vi "OpenTalonDrive.vi"   [LabVIEW 2016]
uses:
  <vilib>/Rock Robotics/WPI/ThirdParty/CanMotor/TalonSRX/WPI_CANTalonSRX_APIControlMode.ctl
  <vilib>/Rock Robotics/WPI/SafetyOutput/WPI_SafetyOutputConfigMenu.ctl
  <vilib>/Rock Robotics/WPI/ThirdParty/CanMotor/TalonSRX/WPI_CANTalonSRX_APIFeedbackSelect.ctl
types:
  T1 = typedef "WPI_CANTalonSRX_APIFeedbackSelect.ctl" = enum16{"Digital Quadrature Encoder", "Analog Potentiometer", "Analog Encoder", "Count on Quad-A (Rising-Edge)", "Count on Quad-A (Falling-Edge)", "CTR Magnetic Enc (Absolute)", "CTR Magnetic Enc (Relative)", "Pulse Width"}
  T2 = typedef "WPI_SafetyOutputConfigMenu.ctl" = enum16{"Enable", "Disable"}
  T3 = typedef "WPI_CANTalonSRX_APIControlMode.ctl" = enum8{"Percent VBus", "Speed", "Position", "Slave", "Unchanged / Invalid", "Voltage Compensation", "Current", "Motion Profile", "Motion Magic"}
  T4 = typedef "WPI_MotorControlDeviceRef.ctl" = cluster{"DeviceStatus":errorcluster, "Type":T5, "PWM":cluster{"PWM Channel":T6, "DeadBand":T7}, "CAN":cluster{"Device Number":u8, "SetOutput VI Ref":variant, "GetOutput VI Ref":variant, "Enable VI Ref":variant, "Disable VI Ref":variant, "Data":variant}, "Invert":bool}
  T5 = typedef "WPI_MotorControlType.ctl" = enum16{"PWM", "CAN"}
  T6 = typedef "FPGA_DIOPWMChannel.ctl" = enum8{"PWM 0", "PWM 1", "PWM 2", "PWM 3", "PWM 4", "PWM 5", "PWM 6", "PWM 7", "PWM 8", "PWM 9", "PWM MXP 0", "PWM MXP 1", "PWM MXP 2", "PWM MXP 3", "PWM MXP 4", "PWM MXP 5", "PWM MXP 6", "PWM MXP 7", "PWM MXP 8", "PWM MXP 9", "Invalid"}
  T7 = typedef "WPI_PWMDeadband.ctl" = cluster{"Name":string, "maxPositivePwm":i32, "minPositivePwm":i32, "centerPwm":i32, "maxNegativePwm":i32, "minNegativePwm":i32, "angularRange":u16}
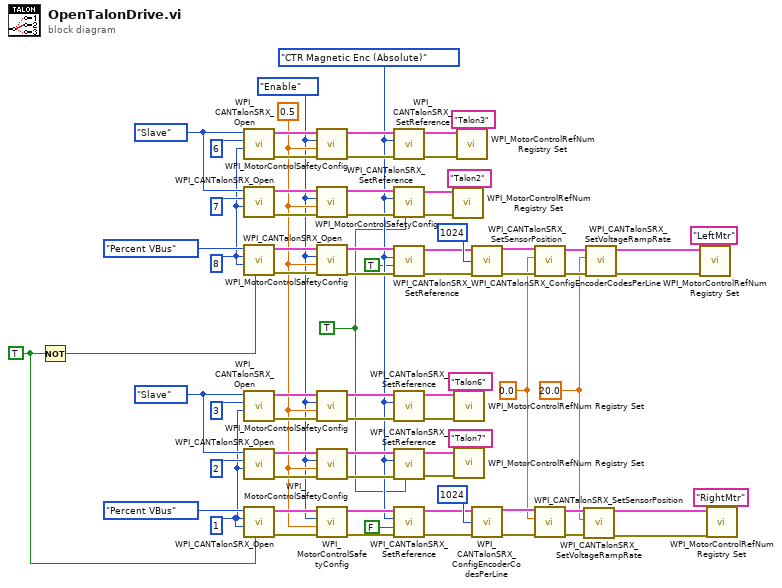
[diagram p0: block diagram]
diagram:
  w5 = 20.0 ("Throttle Ramp Rate (percent/s)")
  w14 = TRUE
  w15 = TRUE
  w30 = WPI_CANTalonSRX_APIFeedbackSelect."CTR Magnetic Enc (Absolute)" ("Feedback Reference")
  w47 = WPI_SafetyOutputConfigMenu."Enable" ("mode")
  w10 = 0.0 ("New Sensor Position")
  w17 = u8 1 ("Device Number")
  w62 = WPI_CANTalonSRX_APIControlMode."Slave" ("Control Mode")
  w48 = 0.5 ("timeout (s)")
  w16 = u8 8 ("Device Number")
  w76 = WPI_CANTalonSRX_APIControlMode."Slave" ("Control Mode")
  n1 = Not(x=w14) -> (.not. x?=w13:bool)
  n2 = call <vilib>:"WPI_CANTalonSRX_Open.vi"("Master Device Number"=w16, "Device Number"=u8 6, "Control Mode"=w76) -> ("error out"=w69:errorcluster, "CAN Talon SRX Ref"=w70:T4)  [unwired: 7 in]
  n3 = call <vilib>:"WPI_CANTalonSRX_Open.vi"("Master Device Number"=w16, "Device Number"=u8 7, "Control Mode"=w76) -> ("error out"=w67:errorcluster, "CAN Talon SRX Ref"=w68:T4)  [unwired: 7 in]
  n4 = call <vilib>:"WPI_CANTalonSRX_Open.vi"("Invert"=w13, "Master Device Number"=w16, "Device Number"=w16, "Control Mode"=WPI_CANTalonSRX_APIControlMode."Percent VBus") -> ("error out"=w71:errorcluster, "CAN Talon SRX Ref"=w72:T4)  [unwired: 6 in]
  n5 = call <vilib>:"WPI_CANTalonSRX_Open.vi"("Master Device Number"=w17, "Device Number"=u8 3, "Control Mode"=w62) -> ("error out"=w55:errorcluster, "CAN Talon SRX Ref"=w56:T4)  [unwired: 7 in]
  n6 = call <vilib>:"WPI_CANTalonSRX_Open.vi"("Master Device Number"=w17, "Device Number"=u8 2, "Control Mode"=w62) -> ("error out"=w53:errorcluster, "CAN Talon SRX Ref"=w54:T4)  [unwired: 7 in]
  n7 = call <vilib>:"WPI_CANTalonSRX_Open.vi"("Invert"=w14, "Master Device Number"=w17, "Device Number"=w17, "Control Mode"=WPI_CANTalonSRX_APIControlMode."Percent VBus") -> ("error out"=w57:errorcluster, "CAN Talon SRX Ref"=w58:T4)  [unwired: 6 in]
  n8 = call <vilib>:"WPI_MotorControlSafetyConfig.vi"("error in (no error)"=w69, "timeout (s)"=w48, "mode"=w47, "MotorControlDevRef"=w70) -> ("error out"=w45:errorcluster, "MotorControlDevRef"=w46:T4)  [unwired: 6 in]
  n9 = call <vilib>:"WPI_MotorControlSafetyConfig.vi"("error in (no error)"=w67, "timeout (s)"=w48, "mode"=w47, "MotorControlDevRef"=w68) -> ("error out"=w43:errorcluster, "MotorControlDevRef"=w44:T4)  [unwired: 6 in]
  n10 = call <vilib>:"WPI_MotorControlSafetyConfig.vi"("error in (no error)"=w71, "timeout (s)"=w48, "mode"=w47, "MotorControlDevRef"=w72) -> ("error out"=w33:errorcluster, "MotorControlDevRef"=w34:T4)  [unwired: 6 in]
  n11 = call <vilib>:"WPI_MotorControlSafetyConfig.vi"("error in (no error)"=w55, "timeout (s)"=w48, "mode"=w47, "MotorControlDevRef"=w56) -> ("error out"=w40:errorcluster, "MotorControlDevRef"=w39:T4)  [unwired: 6 in]
  n12 = call <vilib>:"WPI_MotorControlSafetyConfig.vi"("error in (no error)"=w53, "timeout (s)"=w48, "mode"=w47, "MotorControlDevRef"=w54) -> ("error out"=w42:errorcluster, "MotorControlDevRef"=w41:T4)  [unwired: 6 in]
  n13 = call <vilib>:"WPI_MotorControlSafetyConfig.vi"("error in (no error)"=w57, "timeout (s)"=w48, "mode"=w47, "MotorControlDevRef"=w58) -> ("error out"=w37:errorcluster, "MotorControlDevRef"=w38:T4)  [unwired: 6 in]
  n14 = call <vilib>:"WPI_CANTalonSRX_SetReference.vi"("error in (no error)"=w45, "Feedback Reference"=w30, "CAN Talon SRX Ref"=w46) -> ("error out"=w22:errorcluster, "CAN Talon SRX Ref"=w21:T4)  [unwired: 7 in]
  n15 = call <vilib>:"WPI_CANTalonSRX_SetReference.vi"("Reverse Closed-Loop Output"=w15, "error in (no error)"=w43, "Feedback Reference"=w30, "CAN Talon SRX Ref"=w44) -> ("error out"=w24:errorcluster, "CAN Talon SRX Ref"=w23:T4)  [unwired: 6 in]
  n16 = call <vilib>:"WPI_CANTalonSRX_SetReference.vi"("error in (no error)"=w33, "Reverse Feedback Sensor"=TRUE, "Feedback Reference"=w30, "CAN Talon SRX Ref"=w34) -> ("error out"=w31:errorcluster, "CAN Talon SRX Ref"=w32:T4)  [unwired: 6 in]
  n17 = call <vilib>:"WPI_CANTalonSRX_SetReference.vi"("error in (no error)"=w40, "Feedback Reference"=w30, "CAN Talon SRX Ref"=w39) -> ("error out"=w26:errorcluster, "CAN Talon SRX Ref"=w25:T4)  [unwired: 7 in]
  n18 = call <vilib>:"WPI_CANTalonSRX_SetReference.vi"("Reverse Closed-Loop Output"=w15, "error in (no error)"=w42, "Feedback Reference"=w30, "CAN Talon SRX Ref"=w41) -> ("error out"=w29:errorcluster, "CAN Talon SRX Ref"=w28:T4)  [unwired: 6 in]
  n19 = call <vilib>:"WPI_CANTalonSRX_SetReference.vi"("error in (no error)"=w37, "Reverse Feedback Sensor"=FALSE, "Feedback Reference"=w30, "CAN Talon SRX Ref"=w38) -> ("error out"=w35:errorcluster, "CAN Talon SRX Ref"=w36:T4)  [unwired: 6 in]
  n20 = call <vilib>:"WPI_MotorControlRefNum Registry Set.vi"("error in (no error)"=w24, "refnum name"="Talon2", "MotorControlDevRef"=w23) -> ()  [unwired: 7 in, 2 out]
  n21 = call <vilib>:"WPI_MotorControlRefNum Registry Set.vi"("error in (no error)"=w26, "refnum name"="Talon6", "MotorControlDevRef"=w25) -> ()  [unwired: 7 in, 2 out]
  n22 = call <vilib>:"WPI_MotorControlRefNum Registry Set.vi"("error in (no error)"=w29, "refnum name"="Talon7", "MotorControlDevRef"=w28) -> ()  [unwired: 7 in, 2 out]
  n23 = call <vilib>:"WPI_MotorControlRefNum Registry Set.vi"("error in (no error)"=w22, "refnum name"="Talon3", "MotorControlDevRef"=w21) -> ()  [unwired: 7 in, 2 out]
  n24 = call <vilib>:"WPI_CANTalonSRX_ConfigEncoderCodesPerLine.vi"("CAN Talon SRX Ref"=w32, "Number Encoder Lines\n(Counts Per Rotation)"=u32 1024 ("Number Encoder Lines\n(Counts Per Rotation)"), "error in (no error)"=w31) -> ("CAN Talon SRX Ref"=w64:T4, "error out"=w65:errorcluster)  [unwired: 11 in]
  n25 = call <vilib>:"WPI_CANTalonSRX_ConfigEncoderCodesPerLine.vi"("CAN Talon SRX Ref"=w36, "Number Encoder Lines\n(Counts Per Rotation)"=u32 1024 ("Number Encoder Lines\n(Counts Per Rotation)"), "error in (no error)"=w35) -> ("CAN Talon SRX Ref"=w50:T4, "error out"=w51:errorcluster)  [unwired: 11 in]
  n26 = call <vilib>:"WPI_CANTalonSRX_SetSensorPosition.vi"("error in (no error)"=w65, "New Sensor Position"=w10, "CAN Talon SRX Ref"=w64) -> ("error out"=w6:errorcluster, "CAN Talon SRX Ref"=w7:T4)  [unwired: 7 in]
  n27 = call <vilib>:"WPI_CANTalonSRX_SetSensorPosition.vi"("error in (no error)"=w51, "New Sensor Position"=w10, "CAN Talon SRX Ref"=w50) -> ("error out"=w9:errorcluster, "CAN Talon SRX Ref"=w8:T4)  [unwired: 7 in]
  n28 = call <vilib>:"WPI_CANTalonSRX_SetVoltageRampRate.vi"("error in (no error)"=w9, "Throttle Ramp Rate (percent/s)"=w5, "CAN Talon SRX Ref"=w8) -> ("error out"=w1:errorcluster, "CAN Talon SRX Ref"=w2:T4)  [unwired: 7 in]
  n29 = call <vilib>:"WPI_CANTalonSRX_SetVoltageRampRate.vi"("error in (no error)"=w6, "Throttle Ramp Rate (percent/s)"=w5, "CAN Talon SRX Ref"=w7) -> ("error out"=w4:errorcluster, "CAN Talon SRX Ref"=w3:T4)  [unwired: 7 in]
  n30 = call <vilib>:"WPI_MotorControlRefNum Registry Set.vi"("error in (no error)"=w4, "refnum name"="LeftMtr" ("Ref Name 1"), "MotorControlDevRef"=w3) -> ()  [unwired: 7 in, 2 out]
  n31 = call <vilib>:"WPI_MotorControlRefNum Registry Set.vi"("error in (no error)"=w1, "refnum name"="RightMtr" ("Ref Name 2"), "MotorControlDevRef"=w2) -> ()  [unwired: 7 in, 2 out]
